vi "MainApp.vi"() -> ()   [LabVIEW 2018]
uses:
  TypeDefSERVER/PersonaFisica.ctl
  TypeDefSERVER/ID_REQUEST.ctl
  <vilib>/httpClient/PUTBuffer.vi
  <vilib>/httpClient/LabVIEWHTTPClient.lvlib
panel:
  out "Estado de Verifiacion de credito:":string
  out "Puntos momentaneos":i32
  out "Sujeto a credito?":bool
  in  "VerificarCredito":bool
  in  "ID_SEARCHED":i32(listbox)
  out "Cluster":T1 {"Garantia, patrimonio (valor):" format="$%#_g"; "Utilidad neta" format="$%#_g"; "Flujo de efectivo mensual" format="$%#_g"; "Capital social" format="$%#_g"; "Importe Total" format="$%#_g"}
  # "Puntos momentaneos  == 10"
  # "A;os de antiguedad: 2....4: = 2 puntos momentaneos\n                           mayor4 = 5"
  # "Garantia, patrimonio (valor):  != 0 = + 1 punto momentaneo"
  # ">"
  # "Flujo Anual:  Flujo Efectivo mensual * 12"
  # "10 %Importe total"
  # "Numero de sucursales  > 2    + 2 puntos"
  # "Mayor a 6 puntos = Acesor\n\nEntre 9 y 10 = Se envia correo de acreditacion"
  # "Menor de 6 = Rechazado"
  # "+ 2 puntos"
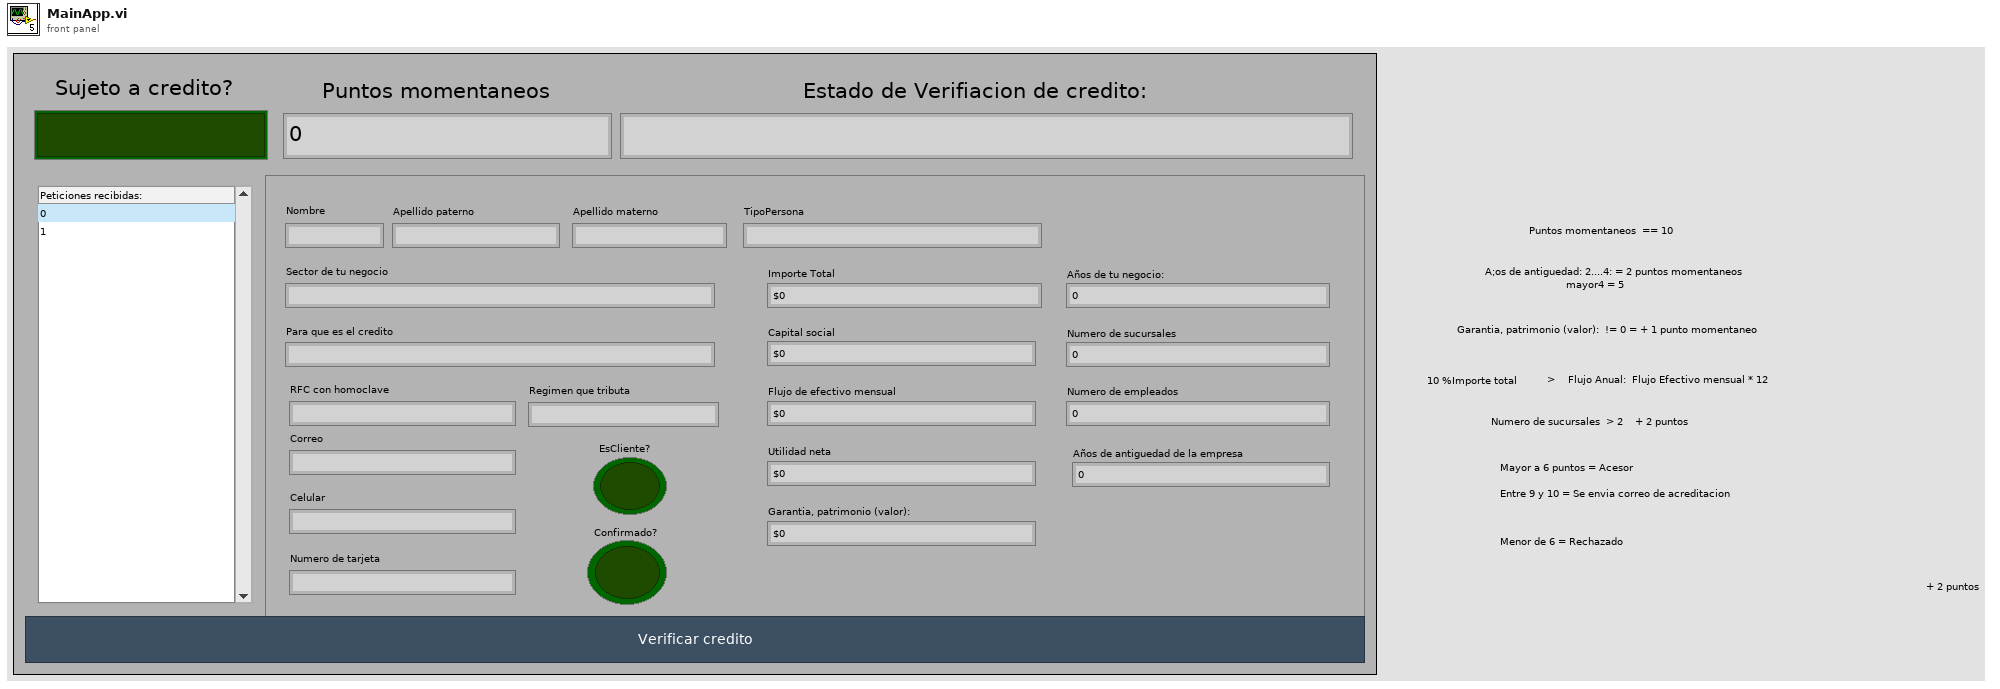
[diagram p1: front panel]
types:
  T1 = typedef "PersonaFisica.ctl" = cluster{"Sector de tu negocio":string, "Para que es el credito":string, "Correo":string, "RFC con homoclave":string, "Nombre":string, "Celular":string, "Apellido materno":string, "Apellido paterno":string, "Años de tu negocio:":i32, "Numero de tarjeta":string, "EsCliente?":bool, "Importe Total":dbl, "Capital social":dbl, "Flujo de efectivo mensual":dbl, "Utilidad neta":dbl, "Garantia, patrimonio (valor):":dbl, "Numero de sucursales":i32, "Numero de empleados":i32, "Años de antiguedad de la empresa":i32, "Regimen que tributa":string, "Confirmado?":bool, "TipoPersona":string}
  T2 = enum16{"init", "wait for a event", "get data", "check if Confirmed?", "close"}
  T3 = cluster{enum16{"init", "wait for a event", "get data", "check if Confirmed?", "close", "ApplyChanges", "SendEmail"}}
  T4 = enum32{"Invalid", "Standard", "Closed", "Hidden", "Minimized", "Maximized"}
  T5 = enum16{"init", "wait for a event", "get data", "check if Confirmed?", "close", "ApplyChanges"}
  T6 = enum16{"init", "wait for a event", "get data", "check if Confirmed?", "close", "ApplyChanges", "SendEmail"}
  T7 = typedef "ID_REQUEST.ctl" = cluster{"ID":i32[]}
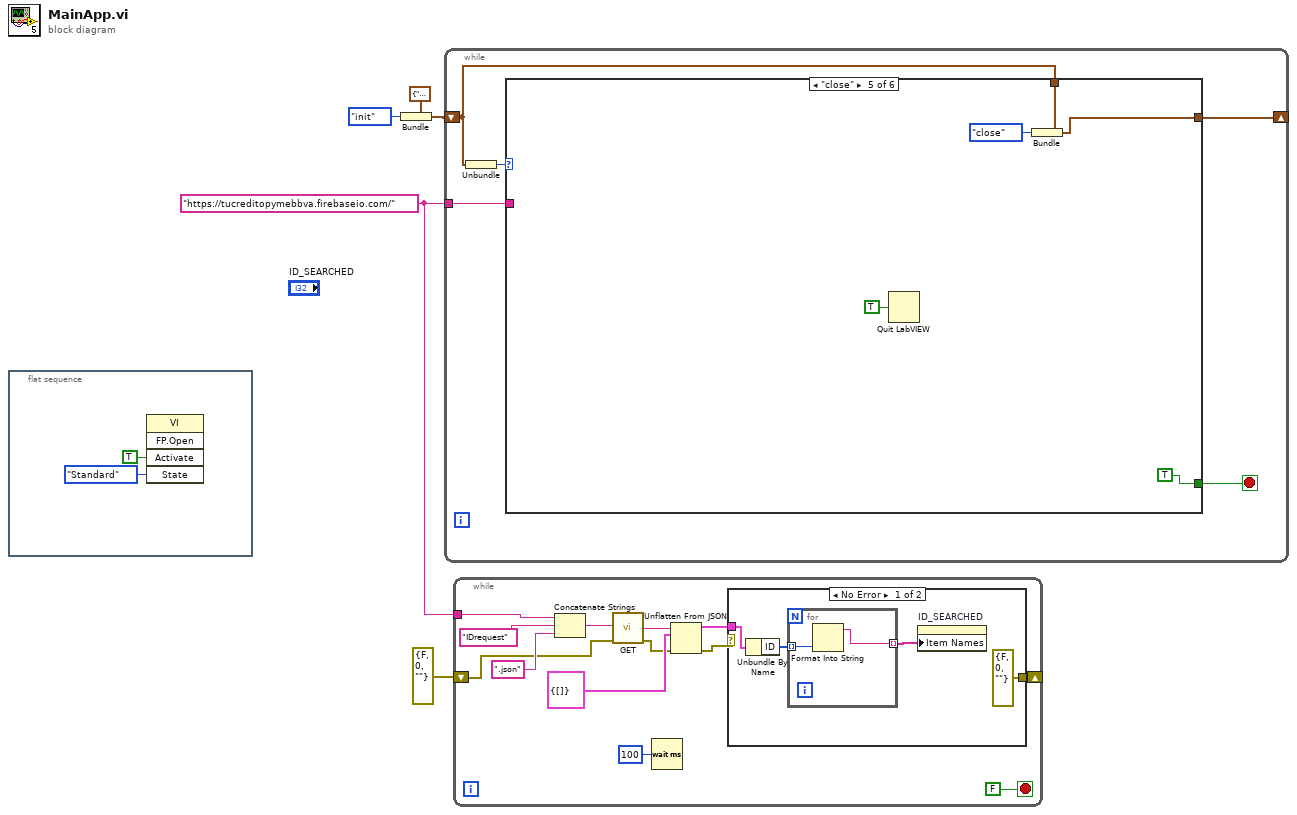
[diagram p0: block diagram]
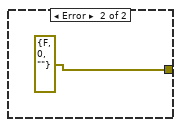
[diagram p2: hidden frame]
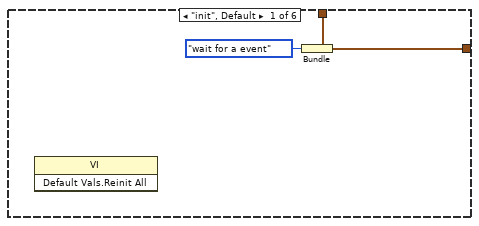
[diagram p3: hidden frame]
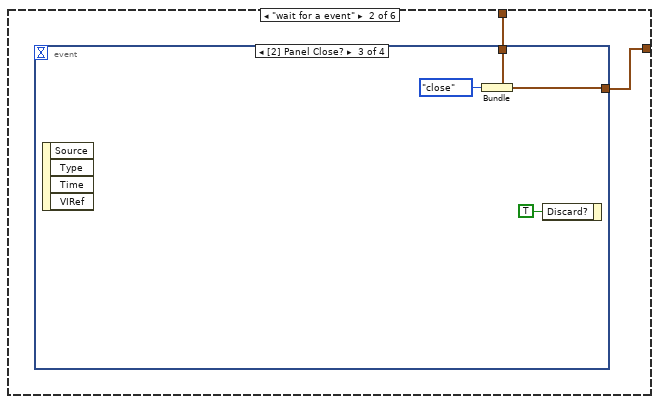
[diagram p4: hidden frame]
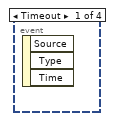
[diagram p5: hidden frame]
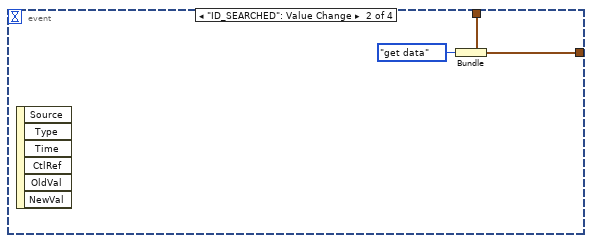
[diagram p6: hidden frame]
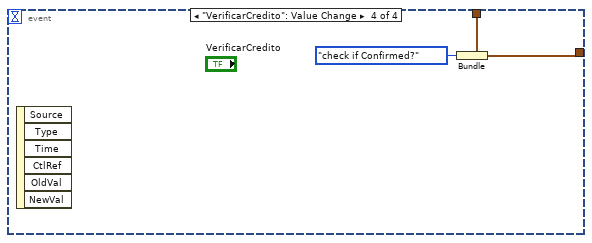
[diagram p7: hidden frame]
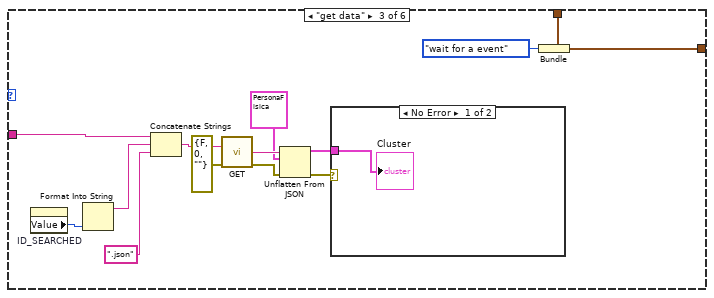
[diagram p8: hidden frame]
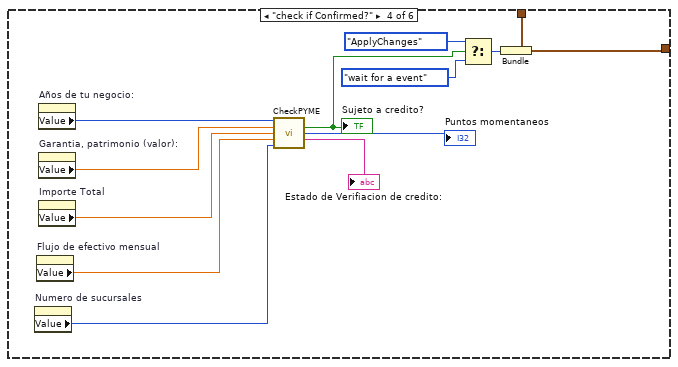
[diagram p10: hidden frame]
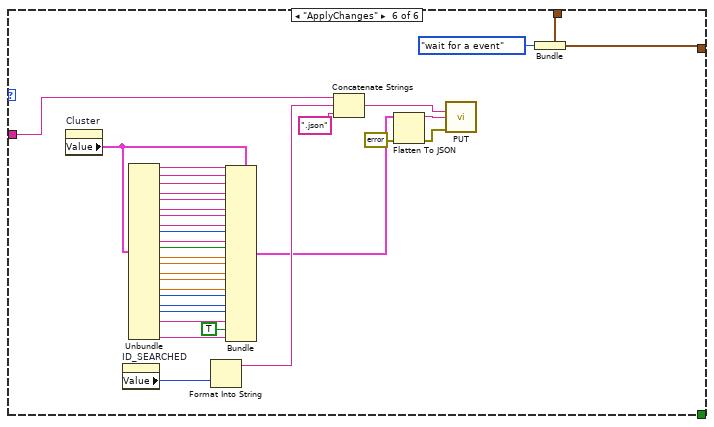
[diagram p11: hidden frame]
diagram:
  w2 = "https://tucreditopymebbva.firebaseio.com/"
  n1 = flat-sequence {
    frame #0 {
      n2 = invoke class="VI" method="FP.Open"("Activate"=TRUE ("Activate?"), "State"=T4."Standard") -> ()  [unwired: 3 in, 5 out]
    }
  }
  n3 = Bundle(cluster=T3 {enum."ApplyChanges"}, T2."init") -> (w3:T3)
  n4 = while {
    shift-right: [w10] -> _
    shift-left: w3 -> [w11]
    tunnel: w2 -> [w9]
    stop <- w8 stop-if-true
    n5 = Unbundle(w11) -> (w12:T6)
    n6 = case shown="\"close\"" w12 {
      tunnel: w11 -> [w15 w17 w41 w55 w60 w63]
      tunnel: [w14 w16 w40 w54 w59 w62] -> w10
      tunnel: w9 -> [_ _ w38 _ _ w71]
      tunnel: [_ _ _ _ TRUE _] -> w8
      frame "init", Default {
        n7 = invoke class="VI" method="Default Vals.Reinit All"() -> ()  [unwired: 3 in, 3 out]
        n8 = Bundle(cluster=w15, T2."wait for a event") -> (w14:T3)
      }
      frame "wait for a event" {
        n9 = event shown="[2] Panel Close?" {
          selector: _ -> [_ _ _ _]
          dyn-events: _ -> [_ _ _ _]
          timeout: _ -> [_ _ _ _]
          tunnel: w17 -> [_ w20 w24 w27]
          tunnel: [_ w18 w23 w26] -> w16
          event Timeout {
            n10 = event-data() -> ()  [unwired: 1 in, 3 out]
          }
          event "ID_SEARCHED": Value Change {
            n11 = event-data() -> ()  [unwired: 1 in, 6 out]
            n12 = Bundle(cluster=w20, T2."get data") -> (w18:T3)
          }
          event Panel Close? {
            n13 = event-data() -> ()  [unwired: 1 in, 4 out]
            n14 = Bundle(cluster=w24, T5."close") -> (w23:T3)
            n15 = event-data("Discard?"=TRUE) -> ()  [unwired: 1 in, 1 out]
          }
          event "VerificarCredito": Value Change {
            n16 = event-data() -> ()  [unwired: 1 in, 6 out]
            n17 = Bundle(cluster=w27, T5."check if Confirmed?") -> (w26:T3)
          }
        }
      }
      frame "get data" {
        n18 = property on="ID_SEARCHED" class="LstBox (strict)"() -> ("Value"=w37:i32)  [unwired: 2 in, 2 out]
        n19 = Format Into String(w37) -> (resulting string=w36:string)  [unwired: 3 in, 1 out]
        n20 = Concatenate Strings(w38, w36, ".json" ("string")) -> (w33:string)
        n21 = call <vilib>:"GET.vi"("url"=w33, "error in (no error)"=errorcluster {"status"=FALSE, "code"=0, "source"=""}) -> ("body"=w34:string, "error out"=w31:errorcluster)  [unwired: 10 in, 2 out]
        n22 = Unflatten From JSON(JSON string=w34, type and defaults=T1 {"Sector de tu negocio"="", "Para que es el credito"="", "Correo"="", "RFC con homoclave"="", "Nombre"="", "Celular"="", "Apellido materno"="", "Apellido paterno"="", "Años de tu negocio:"=0, "Numero de tarjeta"="", "EsCliente?"=FALSE, "Importe Total"=0.0, "Capital social"=0.0, "Flujo de efectivo mensual"=0.0, "Utilidad neta"=0.0, "Garantia, patrimonio (valor):"=0.0, "Numero de sucursales"=0, "Numero de empleados"=0, "Años de antiguedad de la empresa"=0, "Regimen que tributa"="", "Confirmado?"=FALSE, "TipoPersona"=""} ("Cluster"), error in (no error)=w31) -> (value=w28:T1, error out=w29:errorcluster)  [unwired: 4 in]
        n23 = case shown="No Error" w29 {
          tunnel: w28 -> [w42 _]
          frame No Error {
            "Cluster" <- w42
          }
          frame Error {
          }
        }
        n24 = Bundle(cluster=w41, T5."wait for a event") -> (w40:T3)
      }
      frame "check if Confirmed?" {
        n25 = property on="Numero de sucursales" class="DigNum (strict)"() -> ("Value"=w49:i32)  [unwired: 2 in, 2 out]
        n26 = property on="Flujo de efectivo mensual" class="DigNum (strict)"() -> ("Value"=w50:dbl)  [unwired: 2 in, 2 out]
        n27 = property on="Años de tu negocio:" class="DigNum (strict)"() -> ("Value"=w53:i32)  [unwired: 2 in, 2 out]
        n28 = property on="Garantia, patrimonio (valor):" class="DigNum (strict)"() -> ("Value"=w52:dbl)  [unwired: 2 in, 2 out]
        n29 = property on="Importe Total" class="DigNum (strict)"() -> ("Value"=w51:dbl)  [unwired: 2 in, 2 out]
        n30 = call "CheckPYME.vi"("Anos de tu negocio"=w53, "Garantia"=w52, "Importe total"=w51, "Flujo de efectivo mensual"=w50, "Numero de sucursales"=w49) -> ("Sujeto a credito?"=w43:bool, "Puntos momentaneos"=→"Puntos momentaneos":i32, "Status"=→"Estado de Verifiacion de credito:":string)  [unwired: 8 in]
        "Sujeto a credito?" <- w43
        n31 = Select(t=T5."ApplyChanges", s=w43, f=T5."wait for a event") -> (s? t:f=w46:T5)
        n32 = Bundle(cluster=w55, w46) -> (w54:T3)
      }
      frame "close" {
        n33 = Quit LabVIEW(quit? (T)=TRUE) -> ()
        n34 = Bundle(cluster=w60, T5."close") -> (w59:T3)
      }
      frame "ApplyChanges" {
        n35 = property on="Cluster" class="Clust (strict)"() -> ("Value"=w95:T1)  [unwired: 2 in, 2 out]
        n36 = property on="ID_SEARCHED" class="LstBox (strict)"() -> ("Value"=w72:i32)  [unwired: 2 in, 2 out]
        n37 = Unbundle(w95) -> ("Sector de tu negocio"=w94:string, "Para que es el credito"=w93:string, "Correo"=w92:string, "RFC con homoclave"=w91:string, "Nombre"=w90:string, "Celular"=w89:string, "Apellido materno"=w88:string, "Apellido paterno"=w87:string, "Años de tu negocio:"=w86:i32, "Numero de tarjeta"=w85:string, "EsCliente?"=w84:bool, "Importe Total"=w83:dbl, "Capital social"=w82:dbl, "Flujo de efectivo mensual"=w81:dbl, "Utilidad neta"=w80:dbl, "Garantia, patrimonio (valor):"=w79:dbl, "Numero de sucursales"=w78:i32, "Numero de empleados"=w77:i32, "Años de antiguedad de la empresa"=w76:i32, "Regimen que tributa"=w75:string, "TipoPersona"=w74:string)  [unwired: 1 out]
        n38 = Format Into String(w72) -> (resulting string=w70:string)  [unwired: 3 in, 1 out]
        n39 = Bundle(cluster=w95, "Sector de tu negocio"=w94, "Para que es el credito"=w93, "Correo"=w92, "RFC con homoclave"=w91, "Nombre"=w90, "Celular"=w89, "Apellido materno"=w88, "Apellido paterno"=w87, "Años de tu negocio:"=w86, "Numero de tarjeta"=w85, "EsCliente?"=w84, "Importe Total"=w83, "Capital social"=w82, "Flujo de efectivo mensual"=w81, "Utilidad neta"=w80, "Garantia, patrimonio (valor):"=w79, "Numero de sucursales"=w78, "Numero de empleados"=w77, "Años de antiguedad de la empresa"=w76, "Regimen que tributa"=w75, "Confirmado?"=TRUE, "TipoPersona"=w74) -> (w68:T1)
        n40 = Concatenate Strings(w71, w70, ".json" ("string")) -> (w64:string)
        n41 = Flatten To JSON(anything=w68, error in (no error)=errorcluster {"status"=FALSE, "code"=0, "source"=""}) -> (JSON string=w67:string, 11:w66:errorcluster)  [unwired: 1 in]
        n42 = call-poly <vilib>:"PUT.vi"("url"=w64, "buffer"=w67, "error in (no error)"=w66) -> ()  [unwired: 9 in, 4 out]
        n43 = Bundle(cluster=w63, T6."wait for a event") -> (w62:T3)
      }
    }
  }
  n44 = while {
    tunnel: w2 -> [w108]
    shift-right: [w98] -> _
    shift-left: errorcluster {"status"=FALSE, "code"=0, "source"=""} ("error constant") -> [w101]
    stop <- FALSE stop-if-true
    n45 = Concatenate Strings(w108, "IDrequest" ("string"), ".json" ("string")) -> (w105:string)
    n46 = call <vilib>:"GET.vi"("url"=w105, "error in (no error)"=w101) -> ("body"=w104:string, "error out"=w102:errorcluster)  [unwired: 10 in, 2 out]
    n47 = Wait (ms)(milliseconds to wait=u32 100) -> ()  [unwired: 1 out]
    n48 = Unflatten From JSON(JSON string=w104, type and defaults=T7 {"ID"=[]} ("Cluster"), error in (no error)=w102) -> (value=w99:T7, error out=w100:errorcluster)  [unwired: 4 in]
    n49 = case shown="No Error" w100 {
      tunnel: w99 -> [w111 _]
      tunnel: [errorcluster {"status"=FALSE, "code"=0, "source"=""} ("error constant") errorcluster {"status"=FALSE, "code"=0, "source"=""} ("error constant")] -> w98
      frame No Error {
        n50 = Unbundle By Name(w111) -> ("ID"=w110:i32[])
        n51 = for {
          tunnel: w110 -> [w114] mode=indexing
          tunnel: [w113] -> w109 mode=indexing
          n52 = Format Into String(w114) -> (resulting string=w113:string)  [unwired: 3 in, 1 out]
        }
        n53 = property on="ID_SEARCHED" class="LstBox (strict)"("Item Names"=w109) -> ()  [unwired: 2 in, 2 out]
      }
      frame Error {
      }
    }
  }
